vi "TestStand_Builder ( Test-Build ).vi"(8 "error out":errorcluster, 9 "Working_Dir":path, 10 "Test_ID":string="Test\r\n", 11 "Test_Case":string="\nPrecondition:\nPC_1. Wait.Sec(Delay=2) // Wait for Sec\n\nTestProcedure:\nTP_1. Wait.mSec(Delay=1000)  //Waits for ms\n\nReset:\nRST_1. Wait.Sec(Delay=2)  //Waits for sec\r\n") -> (0 "error out 2":errorcluster)   [LabVIEW 2018, in "TestStand_Control.lvlib"]
uses:
  TestStand_Control.lvlib
  Module_Controls/TestStand ( KWD_Info ).ctl
  XML_Library/XML.lvclass
  XML_Library/XML ( Clone and Append Single Input ).vi
  XML_Library/XML ( Set Node Value Single Input ).vi
  XML_Library/XML ( Set Node Value Multiple Inputs ).vi
  XML_Library/XML ( Delete Node Value Single Input ).vi
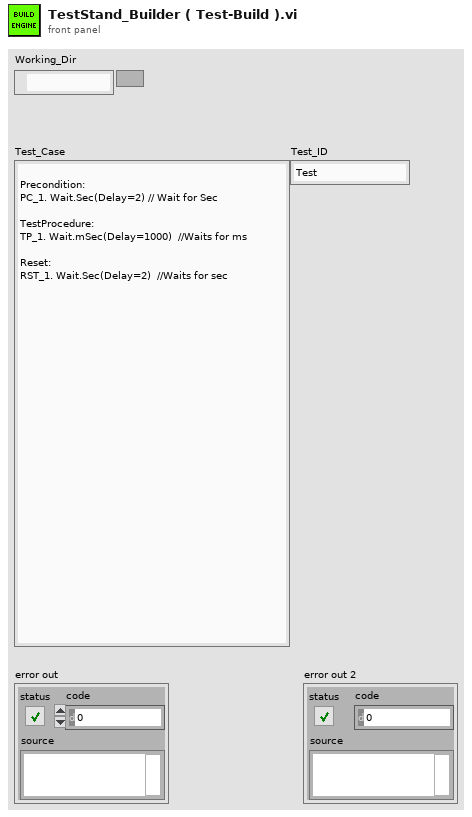
[diagram p1: front panel]
types:
  T1 = enum32{"Invalid", "Standard", "Closed", "Hidden", "Minimized", "Maximized"}
  T2 = enum32{"invalid app kind", "Development System", "Run Time System", "Student Edition", "Embedded LabVIEW", "Evaluation", "Custom"}
  T3 = typedef "TestStand ( KWD_Info ).ctl" = cluster{"Keyword_Name":string, "Keyword_Path":path, "Test_Case":string, "Test_Case Comment":string, "Kwd_Found":bool, "Keyword_Parameters":string}
  T4 = cluster{"Core":cluster{"Current VI Reference":refnum<vi>, "Close Panel on Exit?":bool}, "Test_Case":string, "Test_ID":string, "PreCondition":T3[], "TestProcedure":T3[], "Reset":T3[], "XML":refnum<class "XML.lvclass">}
  T5 = cluster{"Current VI Reference":refnum<vi>, "Close Panel on Exit?":bool}
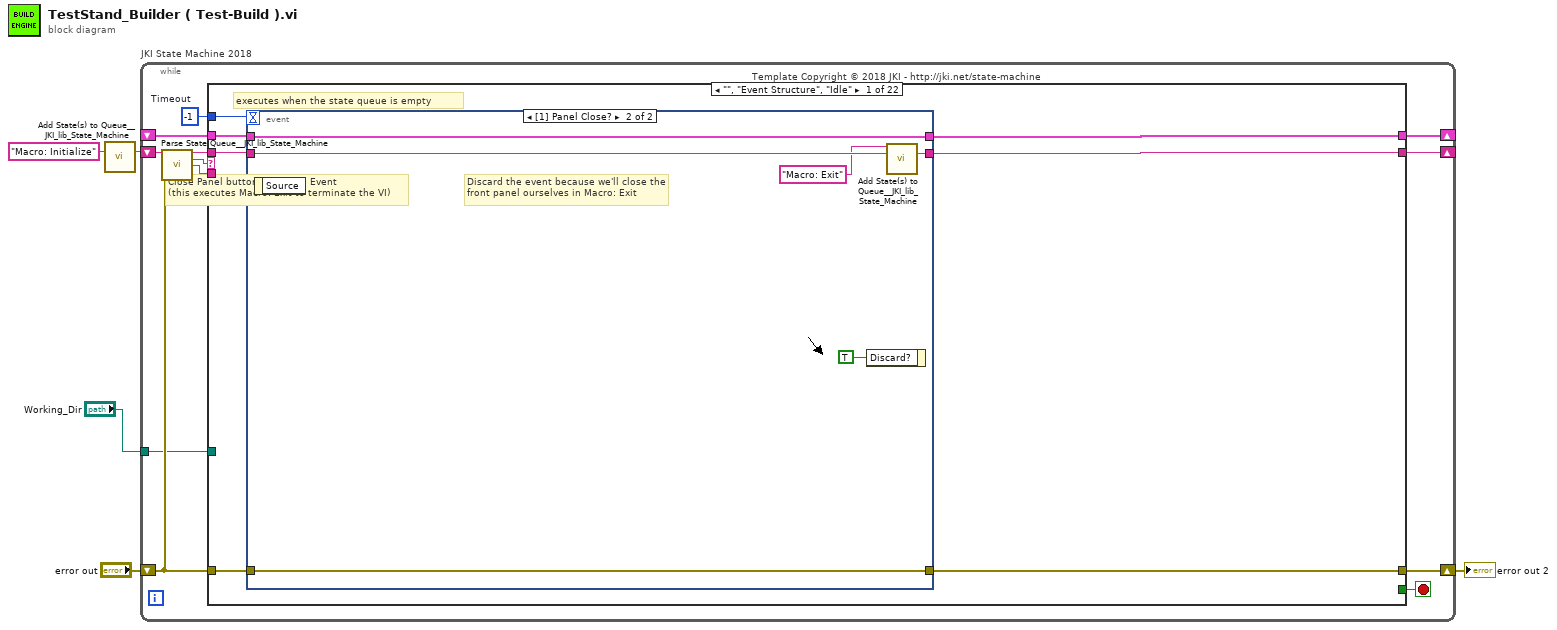
[diagram p0: block diagram]
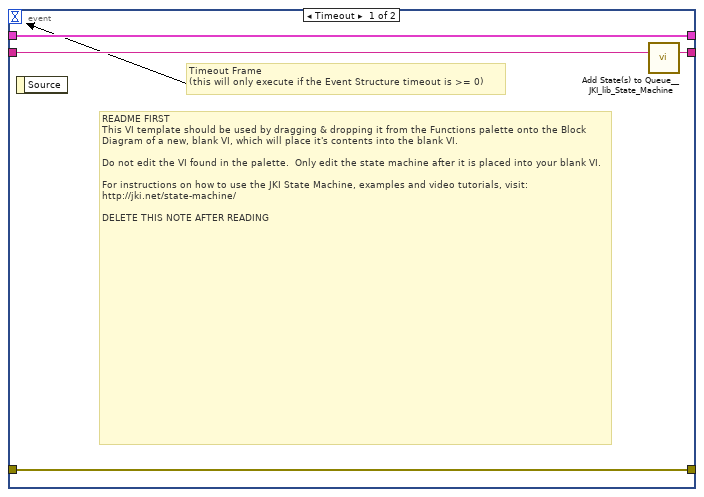
[diagram p2: hidden frame]
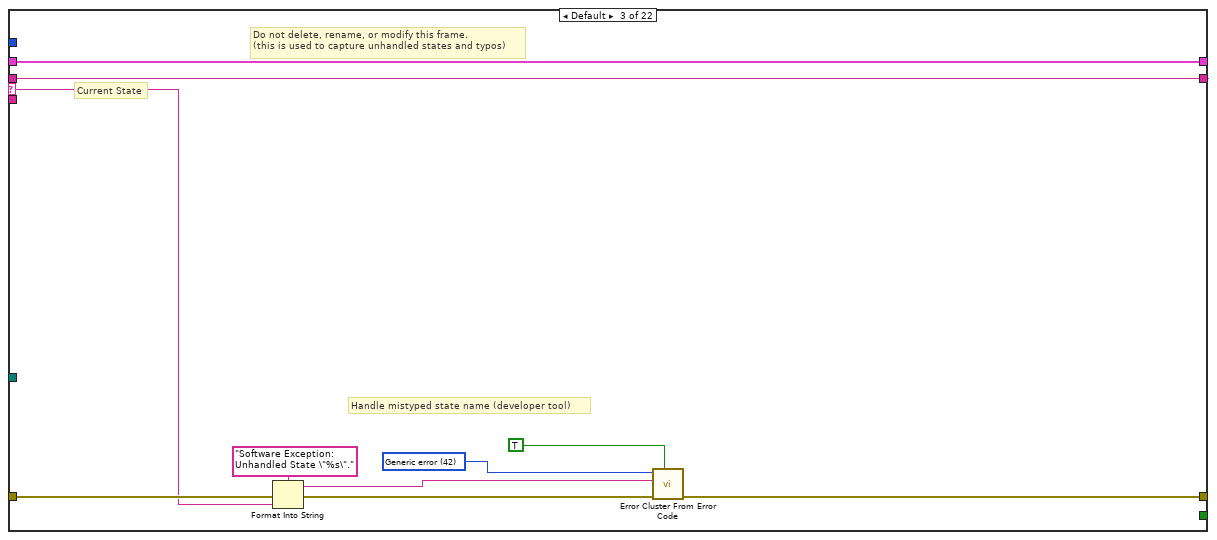
[diagram p4: hidden frame]
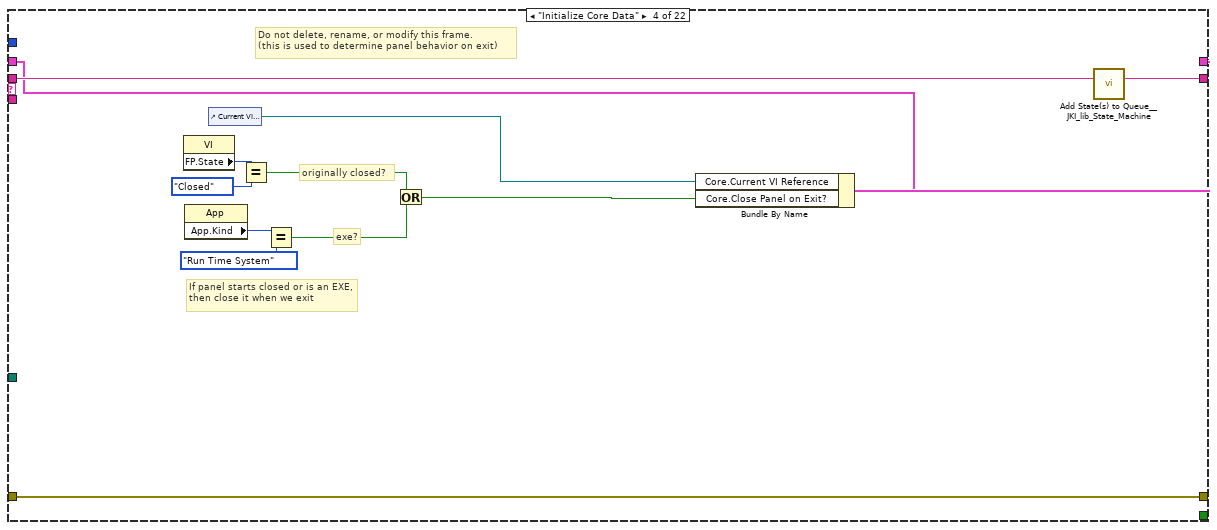
[diagram p5: hidden frame]
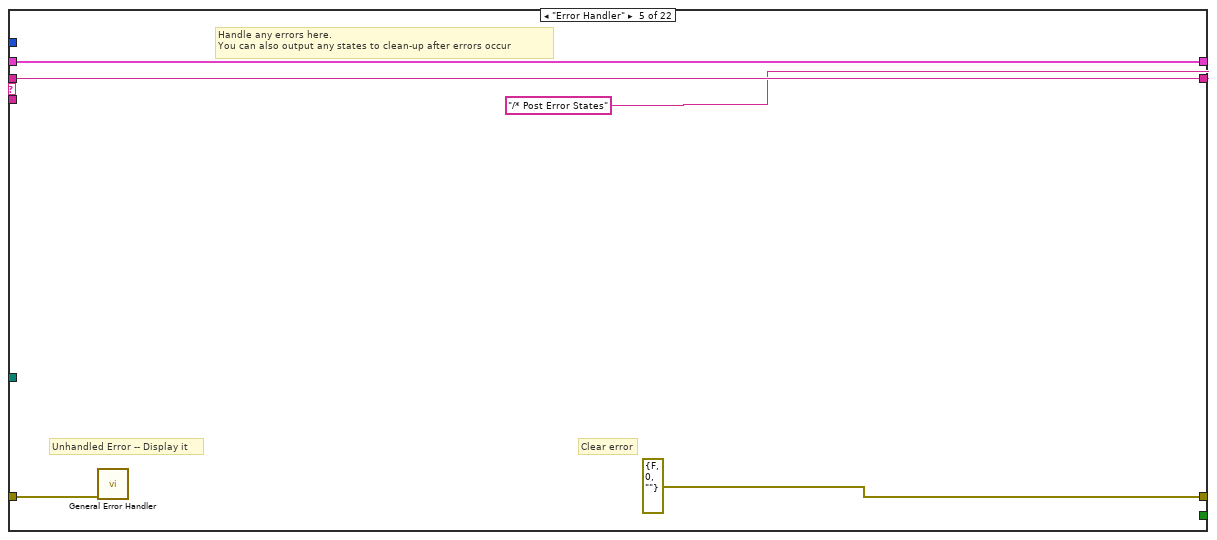
[diagram p6: hidden frame]
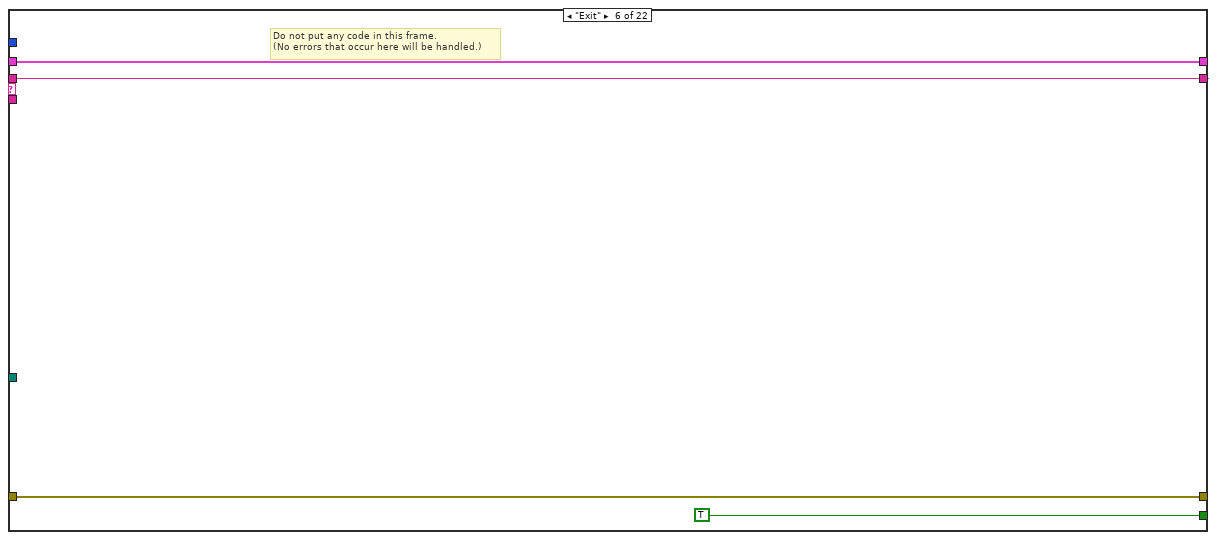
[diagram p7: hidden frame]
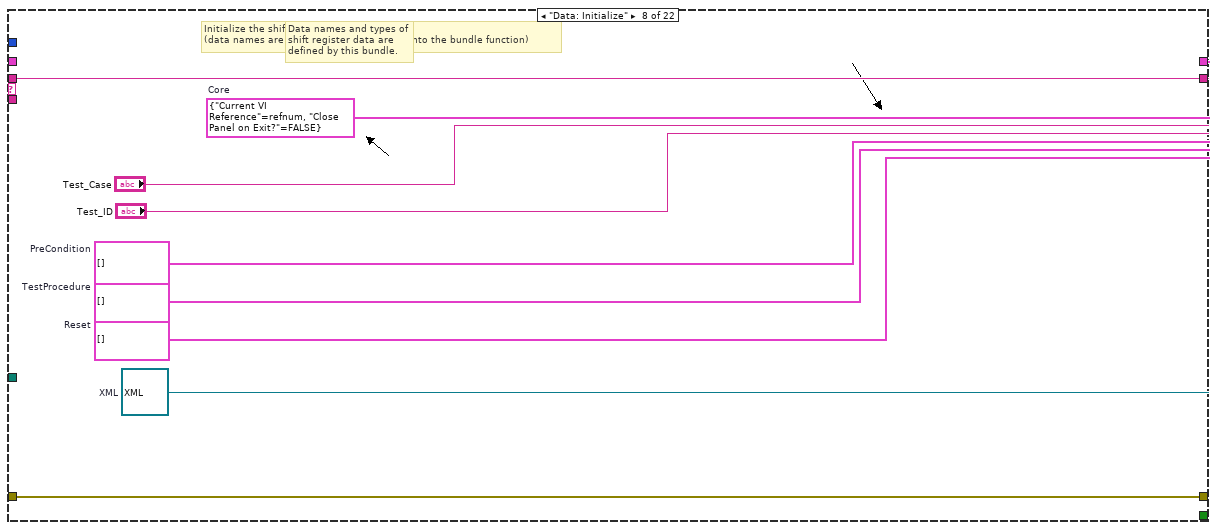
[diagram p9: hidden frame]
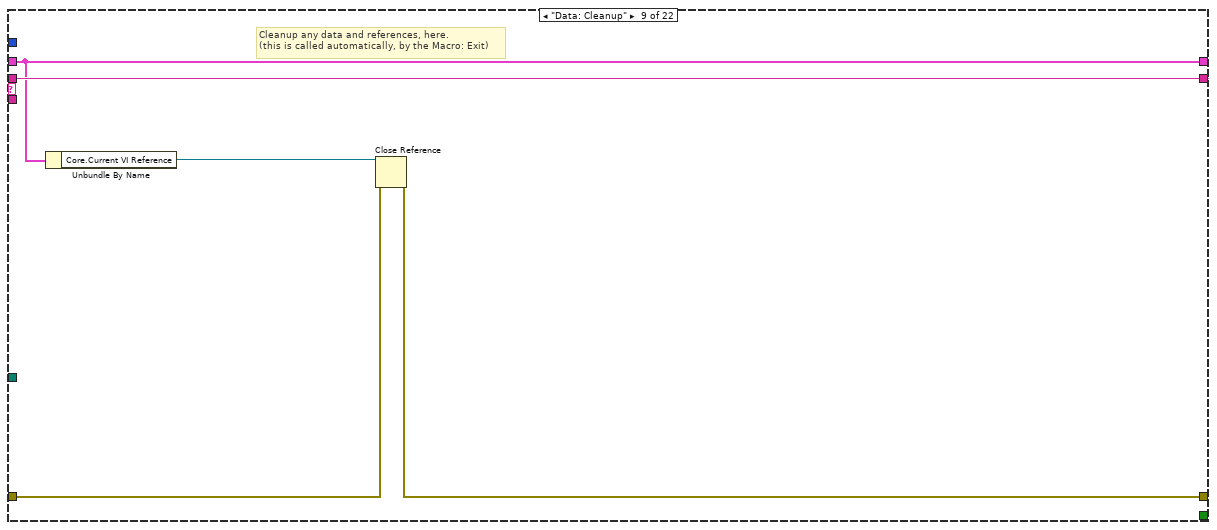
[diagram p10: hidden frame]
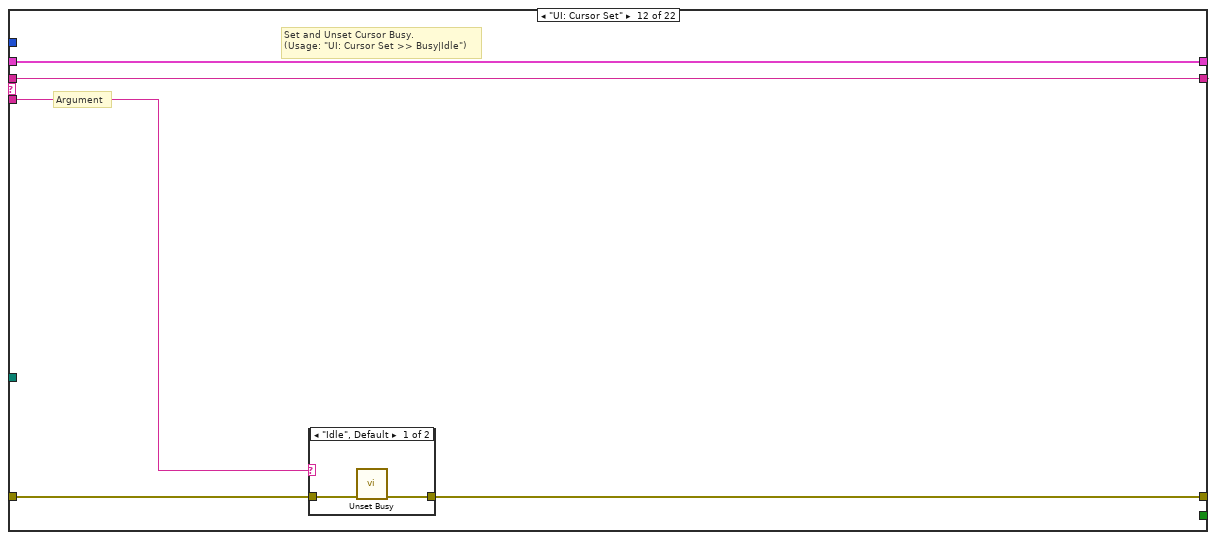
[diagram p13: hidden frame]
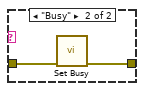
[diagram p14: hidden frame]
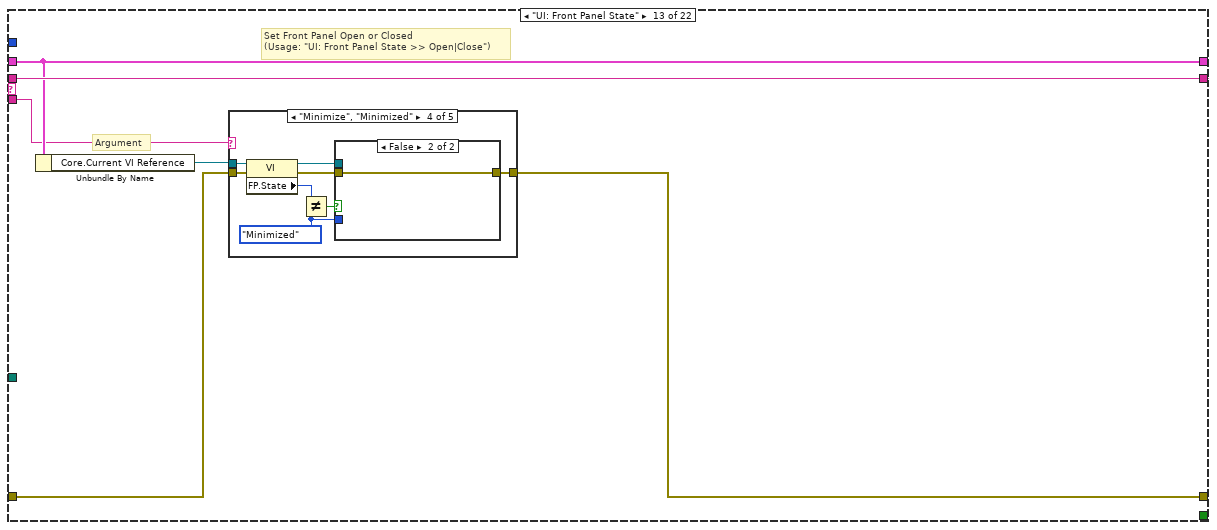
[diagram p15: hidden frame]
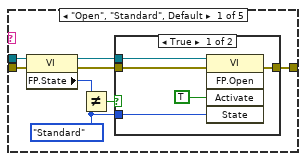
[diagram p16: hidden frame]
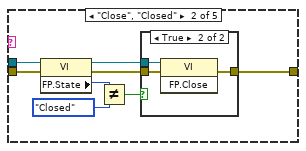
[diagram p18: hidden frame]
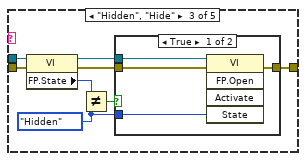
[diagram p20: hidden frame]
diagram:
  n1 = call <vilib>:"Add State(s) to Queue__JKI_lib_State_Machine.vi"("State(s) in (\"\")"="Macro: Initialize") -> ("States Out"=w5:string)  [unwired: 14 in]
  n2 = while "JKI State Machine 2018" {
    shift-right: [w10] -> _
    shift-left: _ -> [w9]
    shift-right: [w13] -> w2
    shift-left: "error out" -> [w7]
    shift-right: [w12] -> _
    shift-left: w5 -> [w14]
    tunnel: "Working_Dir" -> [w6]
    stop <- w11 stop-if-true
    w8 = -1  # Timeout
    # "Template Copyright © 2018 JKI - http://jki.net/state-machine"
    n3 = call <vilib>:"Parse State Queue__JKI_lib_State_Machine.vi"("State Queue"=w14, "Error In (no error)"=w7) -> ("Remaining States"=w16:string, "Current State"=w17:string, "Arguments"=w15:string)  [unwired: 11 in]
    n4 = case shown="\"\", \"Event Structure\", \"Idle\"" w17 {
      selector: w17 -> [_ _ w39 _ _ _ _ _ _ _ _ _ _ _ _ _ _ _ _ w241 _ _]
      tunnel: w16 -> [w24 w38 w43 w62 w68 w73 w77 w88 w94 w98 w102 w108 w119 w188 w193 w203 w207 w218 w230 w243 w344 w367]
      tunnel: w15 -> [_ _ _ _ _ _ _ _ _ _ _ w103 w113 _ _ _ _ _ _ _ _ _]
      tunnel: w9 -> [w22 w35 w41 w55 w65 w71 w74 _ w89 w95 w100 w106 w115 w185 w190 w200 w204 w214 w228 w238 w333 w363]
      tunnel: [w21 w36 w45 w59 errorcluster {"status"=FALSE, "code"=0, "source"=""} ("error out") w70 w75 w85 w90 w96 w99 w104 w116 w186 w191 w201 w205 w216 w225 w235 w324 w359] -> w13
      tunnel: w7 -> [w20 w36 w44 w59 w64 w70 w75 w85 w91 w96 w99 w105 w117 w186 w191 w201 w205 w216 w226 w236 w334 w360]
      tunnel: [w23 w37 w42 w61 w67 w72 w76 w87 w93 w97 w101 w107 w118 w187 w192 w202 w206 w217 w229 w242 w343 w366] -> w12
      tunnel: [_ _ _ _ _ TRUE _ _ _ _ _ _ _ _ _ _ _ _ _ _ _ _] -> w11
      tunnel: [w19 w35 w41 w60 w65 w71 w74 w86 w89 w95 w100 w106 w115 w185 w190 w200 w204 w213 w224 w233 w329 w363] -> w10
      tunnel: w8 -> [w18 _ _ _ _ _ _ _ _ _ _ _ _ _ _ _ _ _ _ _ _ _]
      tunnel: w6 -> [_ _ _ _ _ _ _ _ _ _ _ _ _ _ _ _ _ w208 w221 _ _ w356]
      frame "", "Event Structure", "Idle" {
        # "executes when the state queue is empty"
        n5 = event shown="[1] Panel Close?" {
          selector: _ -> [_ _]
          dyn-events: _ -> [_ _]
          timeout: w18 -> [_ _]
          tunnel: w24 -> [w28 w34]
          tunnel: [w27 w33] -> w23
          tunnel: w22 -> [w25 w31]
          tunnel: [w26 w32] -> w21
          tunnel: w20 -> [w26 w32]
          tunnel: [w25 w31] -> w19
          event Timeout {
            # "README FIRST\nThis VI template should be used by dragging & dropping it from the Functions palette onto the Block Diagram of a new, blank VI, which will place it's contents into the blank VI.\n\nDo not edit the VI found in the palette.  Only edit the state machine after it is placed into your blank VI.\n\nFor instructions on how to use the JKI State Machine, examples and video tutorials, visit:\nhttp://jki.net/state-machine/\n\nDELETE THIS NOTE AFTER READING"
            # "Timeout Frame\n(this will only execute if the Event Structure timeout is >= 0)"
            n6 = event-data() -> ()  [unwired: 1 in, 1 out]
            n7 = call <vilib>:"Add State(s) to Queue__JKI_lib_State_Machine.vi"("State(s) in (\"\")"=w28) -> ("States Out"=w27:string)  [unwired: 14 in]
          }
          event Panel Close? {
            # "Discard the event because we'll close the front panel ourselves in Macro: Exit"
            # "Close Panel button (pressed) Event\n(this executes Macro: Exit to terminate the VI)"
            n8 = event-data() -> ()  [unwired: 1 in, 1 out]
            n9 = event-data("Discard?"=TRUE) -> ()  [unwired: 1 in, 1 out]
            n10 = call <vilib>:"Add State(s) to Queue__JKI_lib_State_Machine.vi"("State(s) in Front (\"\")"="Macro: Exit", "State(s) in (\"\")"=w34) -> ("States Out"=w33:string)  [unwired: 13 in]
          }
        }
      }
      frame "---------- Core ----------" {
        # "Do not put any code in this frame.\n(it is a separator no-op)"
        n11 = call <vilib>:"Add State(s) to Queue__JKI_lib_State_Machine.vi"("State(s) in (\"\")"=w38) -> ("States Out"=w37:string)  [unwired: 14 in]
      }
      frame Default {
        w48 = 42 items=["No error", "Argument error", "Memory is full", "Out of zone", "End of file", "File already open", "Generic file I/O error", "File not found", "File permission error", "Disk is full", "Duplicate path", "Too many files open", "System feature not enabled", "Resource file not found", "Cannot add resource", "Resource not found", "Image not found", "Image memory error", "Pen does not exist", "Config type invalid", "Config token not found", "Config parse error", "Config memory error", "Bad external code format", "Bad external code offset", "External code not present", "Null window", "Destroy window error", "Null menu", "Print aborted", "Bad print record", "Print driver error", "Windows error during printing", "Memory error during printing", "Print dialog error", "Generic print error", "Invalid device refnum", "Device not found", "Device parameter error", "Device unit error", "Cannot open device", "Device call aborted", "Generic error", "Cancelled by user", "Object ID too low", "Object ID too high", "Object not in heap", "Unknown heap", "Unknown object (invalid DefProc)", "Unknown object (DefProc not in table)", "Message out of range", "Invalid (null) method", "Unknown message", "Manager call not supported", "Bad address", "Network operation in progress", "Network operation timed out", "Connection is busy", "Network attribute not supported", "Network error", "Address in use", "System out of memory", "Connection aborted", "Connection refused", "Not connected", "Already connected", "Connection closed", "Initialization error (interapplication manager)", "Bad occurrence", "Wait on unbound occurrence handler", "Occurrence queue overflow", "Datalog type conflict", "Unused", "Unrecognized type (interapplication manager)", "Memory corrupt", "Failed to make temporary DLL", "Old CIN version", "Drag socket not found", "Failed to load drop-object", "Failed to register OLE object", "Failed to release OLE object", "Format specifier type mismatch", "Unknown format specifier", "Too few format specifiers", "Too many format specifiers", "Scan failed", "Newer CIN version", "Error converting to variant", "Runtime menu error", "Password tampered", "Variant attribute not found", "Incompatible variant data type", "Event data is not available", "Event Store is not present", "Occurrence is not found", "Event Queue is not created", "Event info is not available", "Refnum passed is NULL", "Error retrieving Class GUID", "Error retrieving CoClass GUID", "Error retrieving TypeLib GUID.", "Bad built application magic bytes.", "Specific driver is different from the specific driver associated with the Logical Name.", "There is no session opened to the class driver.", "Max Error", "MAX - Error with config objects", "MAX - Error loading configuration", "MAX - Group not supported"]
        # "Current State"
        # "Do not delete, rename, or modify this frame.\n(this is used to capture unhandled states and typos)"
        # "Handle mistyped state name (developer tool)"
        n12 = Format Into String(format string="Software Exception: Unhandled State \"%s\"." ("message"), error in=w44, w39) -> (resulting string=w47:string, error out=w46:errorcluster)  [unwired: 1 in]
        n13 = call <vilib>:"Error Cluster From Error Code.vi"("show call chain? (False)"=TRUE, "error in (no error)"=w46, "error message (\"\")"=w47, "error code (0)"=w48) -> ("error out"=w45:errorcluster)  [unwired: 5 in]
        n14 = call <vilib>:"Add State(s) to Queue__JKI_lib_State_Machine.vi"("State(s) in (\"\")"=w43) -> ("States Out"=w42:string)  [unwired: 14 in]
      }
      frame "Initialize Core Data" {
        # "Do not delete, rename, or modify this frame.\n(this is used to determine panel behavior on exit)"
        # "originally closed?"
        # "exe?"
        # "If panel starts closed or is an EXE, then close it when we exit"
        n15 = property class="VI"() -> ("FP.State"=w52:T1)  [unwired: 2 in, 2 out]
        n16 = property class="App"() -> ("App.Kind"=w58:T2)  [unwired: 2 in, 2 out]
        n17 = control-ref of="Current VI Reference"() -> (w53:refnum<vi>)
        n18 = Equal?(x=w52, y=T1."Closed" ("Front Panel Window:State")) -> (x = y?=w50:bool)
        n19 = Equal?(x=w58, y=T2."Run Time System" ("Application:Kind")) -> (x = y?=w56:bool)
        n20 = Or(x=w50, y=w56) -> (x .or. y?=w54:bool)
        n21 = Bundle By Name(cluster=w55, "Core.Current VI Reference"=w53, "Core.Close Panel on Exit?"=w54) -> (w60:T4)
        n22 = call <vilib>:"Add State(s) to Queue__JKI_lib_State_Machine.vi"("State(s) in (\"\")"=w62) -> ("States Out"=w61:string)  [unwired: 14 in]
      }
      frame "Error Handler" {
        # "Unhandled Error -- Display it"
        # "Handle any errors here.\nYou can also output any states to clean-up after errors occur"
        # "Clear error"
        n23 = call <vilib>:"General Error Handler.vi"("error in (no error)"=w64) -> ()  [unwired: 10 in, 5 out]
        n24 = call <vilib>:"Add State(s) to Queue__JKI_lib_State_Machine.vi"("State(s) in Front (\"\")"="/* Post Error States", "State(s) in (\"\")"=w68) -> ("States Out"=w67:string)  [unwired: 13 in]
      }
      frame "Exit" {
        # "Do not put any code in this frame.\n(No errors that occur here will be handled.)"
        n25 = call <vilib>:"Add State(s) to Queue__JKI_lib_State_Machine.vi"("State(s) in (\"\")"=w73) -> ("States Out"=w72:string)  [unwired: 14 in]
      }
      frame "---------- Data ----------" {
        # "Do not put any code in this frame.\n(It is a separator no-op. You can make a copy of this frame to create a new Data frame)"
        n26 = call <vilib>:"Add State(s) to Queue__JKI_lib_State_Machine.vi"("State(s) in (\"\")"=w77) -> ("States Out"=w76:string)  [unwired: 14 in]
      }
      frame "Data: Initialize" {
        w80 = refnum<class "XML.lvclass"> refnum  # XML
        w81 = T3[] []  # Reset
        w82 = T3[] []  # TestProcedure
        w78 = T3[] []  # PreCondition
        w84 = T5 {"Current VI Reference"=refnum, "Close Panel on Exit?"=FALSE}  # Core
        # "Data names and types of shift register data are defined by this bundle."
        # "Initialize the shift-register data, here.\n(data names are defined by what you wire into the bundle function)"
        n27 = call <vilib>:"Add State(s) to Queue__JKI_lib_State_Machine.vi"("State(s) in (\"\")"=w88) -> ("States Out"=w87:string)  [unwired: 14 in]
        n28 = Bundle("Core"=w84, "Test_Case"="Test_Case", "Test_ID"="Test_ID", "PreCondition"=w78, "TestProcedure"=w82, "Reset"=w81, "XML"=w80) -> (w86:T4)  [unwired: 1 in]
      }
      frame "Data: Cleanup" {
        # "Cleanup any data and references, here.\n(this is called automatically, by the Macro: Exit)"
        n29 = Unbundle By Name(w89) -> ("Core.Current VI Reference"=w92:refnum<vi>)
        n30 = Close Reference(reference=w92, error in (no error)=w91) -> (error out=w90:errorcluster)
        n31 = call <vilib>:"Add State(s) to Queue__JKI_lib_State_Machine.vi"("State(s) in (\"\")"=w94) -> ("States Out"=w93:string)  [unwired: 14 in]
      }
      frame "---------- UI ----------" {
        # "Do not put any code in this frame.\n(It is a separator no-op. You can make a copy of this frame to create a new UI frame)"
        n32 = call <vilib>:"Add State(s) to Queue__JKI_lib_State_Machine.vi"("State(s) in (\"\")"=w98) -> ("States Out"=w97:string)  [unwired: 14 in]
      }
      frame "UI: Initialize" {
        # "Initialize the User Interface, here.\n(this is called automatically, by the Macro: Init)"
        n33 = call <vilib>:"Add State(s) to Queue__JKI_lib_State_Machine.vi"("State(s) in (\"\")"=w102) -> ("States Out"=w101:string)  [unwired: 14 in]
      }
      frame "UI: Cursor Set" {
        # "Argument"
        # "Set and Unset Cursor Busy.\n(Usage: \"UI: Cursor Set >> Busy|Idle\")"
        n34 = case shown="\"Idle\", Default" w103 {
          tunnel: w105 -> [w110 w112]
          tunnel: [w109 w111] -> w104
          frame "Idle", Default {
            n35 = call <vilib>:"Unset Busy.vi"("error in (no error)"=w110) -> ("error out"=w109:errorcluster)  [unwired: 10 in]
          }
          frame "Busy" {
            n36 = call <vilib>:"Set Busy.vi"("error in (no error)"=w112) -> ("error out"=w111:errorcluster)  [unwired: 9 in, 1 out]
          }
        }
        n37 = call <vilib>:"Add State(s) to Queue__JKI_lib_State_Machine.vi"("State(s) in (\"\")"=w108) -> ("States Out"=w107:string)  [unwired: 14 in]
      }
      frame "UI: Front Panel State" {
        # "Argument"
        # "Set Front Panel Open or Closed\n(Usage: \"UI: Front Panel State >> Open|Close\")"
        n38 = Unbundle By Name(w115) -> ("Core.Current VI Reference"=w114:refnum<vi>)
        n39 = case shown="\"Minimize\", \"Minimized\"" w113 {
          tunnel: w117 -> [w125 w140 w151 w164 w177]
          tunnel: [w127 w141 w153 w166 w179] -> w116
          tunnel: w114 -> [w126 w138 w152 w165 w178]
          frame "Open", "Standard", Default {
            w120 = T1."Standard" ("State")
            n40 = property class="VI"(reference=w126, error in=w125) -> (reference out=w123:refnum<vi>, error out=w124:errorcluster, "FP.State"=w122:T1)
            n41 = Not Equal?(x=w122, y=w120) -> (x != y?=w121:bool)
            n42 = case shown="True" w121 {
              tunnel: [w131 w133] -> w127
              tunnel: w124 -> [w130 w133]
              tunnel: w123 -> [w129 _]
              tunnel: w120 -> [w128 _]
              frame True {
                n43 = invoke class="VI" method="FP.Open"(reference=w129, error in=w130, "Activate"=TRUE, "State"=w128) -> (error out=w131:errorcluster)  [unwired: 1 in, 4 out]
              }
              frame False {
              }
            }
          }
          frame "Close", "Closed" {
            n44 = property class="VI"(reference=w138, error in=w140) -> (reference out=w137:refnum<vi>, error out=w139:errorcluster, "FP.State"=w135:T1)
            n45 = Not Equal?(x=w135, y=T1."Closed" ("Front Panel Window:State")) -> (x != y?=w134:bool)
            n46 = case shown="True" w134 {
              tunnel: [w142 w145] -> w141
              tunnel: w139 -> [w142 w144]
              tunnel: w137 -> [_ w143]
              frame False {
              }
              frame True {
                n47 = invoke class="VI" method="FP.Close"(reference=w143, error in=w144) -> (error out=w145:errorcluster)  [unwired: 1 in, 2 out]
              }
            }
          }
          frame "Hidden", "Hide" {
            w146 = T1."Hidden" ("State")
            n48 = property class="VI"(reference=w152, error in=w151) -> (reference out=w149:refnum<vi>, error out=w150:errorcluster, "FP.State"=w148:T1)
            n49 = Not Equal?(x=w148, y=w146) -> (x != y?=w147:bool)
            n50 = case shown="True" w147 {
              tunnel: [w157 w158] -> w153
              tunnel: w150 -> [w156 w158]
              tunnel: w149 -> [w155 _]
              tunnel: w146 -> [w154 _]
              frame True {
                n51 = invoke class="VI" method="FP.Open"(reference=w155, error in=w156, "State"=w154) -> (error out=w157:errorcluster)  [unwired: 2 in, 4 out]
              }
              frame False {
              }
            }
          }
          frame "Minimize", "Minimized" {
            w159 = T1."Minimized" ("State")
            n52 = property class="VI"(reference=w165, error in=w164) -> (reference out=w162:refnum<vi>, error out=w163:errorcluster, "FP.State"=w161:T1)
            n53 = Not Equal?(x=w161, y=w159) -> (x != y?=w160:bool)
            n54 = case shown="False" w160 {
              tunnel: [w170 w171] -> w166
              tunnel: w163 -> [w169 w171]
              tunnel: w162 -> [w168 _]
              tunnel: w159 -> [w167 _]
              frame True {
                n55 = invoke class="VI" method="FP.Open"(reference=w168, error in=w169, "State"=w167) -> (error out=w170:errorcluster)  [unwired: 2 in, 4 out]
              }
              frame False {
              }
            }
          }
          frame "Maximize", "Maximized" {
            w172 = T1."Maximized" ("State")
            n56 = property class="VI"(reference=w178, error in=w177) -> (reference out=w175:refnum<vi>, error out=w176:errorcluster, "FP.State"=w174:T1)
            n57 = Not Equal?(x=w174, y=w172) -> (x != y?=w173:bool)
            n58 = case shown="True" w173 {
              tunnel: [w183 w184] -> w179
              tunnel: w176 -> [w182 w184]
              tunnel: w175 -> [w181 _]
              tunnel: w172 -> [w180 _]
              frame True {
                n59 = invoke class="VI" method="FP.Open"(reference=w181, error in=w182, "State"=w180) -> (error out=w183:errorcluster)  [unwired: 2 in, 4 out]
              }
              frame False {
              }
            }
          }
        }
        n60 = call <vilib>:"Add State(s) to Queue__JKI_lib_State_Machine.vi"("State(s) in (\"\")"=w119) -> ("States Out"=w118:string)  [unwired: 14 in]
      }
      frame "---------- Macro ----------" {
        # "Do not put any code in this frame.\n(It is a separator no-op. You can make a copy of this frame to create a new Macro frame)"
        n61 = call <vilib>:"Add State(s) to Queue__JKI_lib_State_Machine.vi"("State(s) in (\"\")"=w188) -> ("States Out"=w187:string)  [unwired: 14 in]
      }
      frame "Macro: Initialize" {
        w189 = "Data: Initialize\nInitialize Core Data\nUI: Initialize\nUI: Front Panel State >> Minimize\nBuild_Engine: TestCase_KWD"  # Data: Initialize Initialize Core Data UI: Initialize UI: Front Panel State >> Minimize Build_Engine: TestCase_KWD
        # "Initialization Macro\n(This is called once, when the VI starts)"
        n62 = call <vilib>:"Add State(s) to Queue__JKI_lib_State_Machine.vi"("State(s) in Front (\"\")"=w189, "State(s) in (\"\")"=w193) -> ("States Out"=w192:string)  [unwired: 13 in]
      }
      frame "Macro: Exit" {
        # "Exit Macro\n(This is called once, when the VI exits)"
        n63 = Unbundle By Name(w200) -> ("Core.Close Panel on Exit?"=w199:bool)
        n64 = Select(t="UI: Front Panel State >> Close", s=w199, f="") -> (s? t:f=w196:string)
        n65 = call <vilib>:"Add State(s) to Queue__JKI_lib_State_Machine.vi"("State(s) in (\"\")"=w196, "State(s) at Back (\"\")"="Data: Cleanup\nExit") -> ("States Out"=w194:string)  [unwired: 13 in]
        n66 = call <vilib>:"Add State(s) to Queue__JKI_lib_State_Machine.vi"("State(s) in Front (\"\")"=w194, "State(s) in (\"\")"=w203) -> ("States Out"=w202:string)  [unwired: 13 in]
      }
      frame "---------- Build_Engine ----------" {
        # "Your code here.\n(You can make a copy of, or modify, this frame)"
        n67 = call <vilib>:"Add State(s) to Queue__JKI_lib_State_Machine.vi"("State(s) in (\"\")"=w207) -> ("States Out"=w206:string)  [unwired: 14 in]
      }
      frame "Build_Engine: TestCase_KWD" {
        # "Your code here.\n(You can make a copy of, or modify, this frame)"
        n68 = Unbundle By Name(w214) -> ("Test_Case"=w215:string)
        n69 = call "TestStand_Control ( Keyword_TestCase_Linkage ).vi"("Working_Directory"=w208, "Test_Case"=w215) -> ("Reset"=w210:T3[], "TestProcedure"=w211:T3[], "PreCondition"=w212:T3[])  [unwired: 7 in]
        n70 = Bundle By Name(cluster=w214, "PreCondition"=w212, "TestProcedure"=w211, "Reset"=w210) -> (w213:T4)
        n71 = call <vilib>:"Add State(s) to Queue__JKI_lib_State_Machine.vi"("State(s) in Front (\"\")"="Build_Engine: Init" ("State(s) in Front (\"\")"), "State(s) in (\"\")"=w218) -> ("States Out"=w217:string)  [unwired: 13 in]
      }
      frame "Build_Engine: Init" {
        # "Your code here.\n(You can make a copy of, or modify, this frame)"
        n72 = Unbundle By Name(w228) -> ("XML"=w227:refnum<class "XML.lvclass">)
        n73 = Build Path(base path=w221, name or relative path="Template\\Template.seq") -> (appended path=w219:path)
        n74 = call "XML ( Open ).vi"("error in (no error)"=w226, "XML document"=w219, "XML in"=w227) -> ("error out"=w225:errorcluster, "XML out"=w223:refnum<class "XML.lvclass">)  [unwired: 7 in]
        n75 = Bundle By Name(cluster=w228, "XML"=w223) -> (w224:T4)
        n76 = call <vilib>:"Add State(s) to Queue__JKI_lib_State_Machine.vi"("State(s) in Front (\"\")"="Build_Engine: Build_PC" ("State(s) in Front (\"\")"), "State(s) in (\"\")"=w230) -> ("States Out"=w229:string)  [unwired: 13 in]
      }
      frame "Build_Engine: Build_PC", "Build_Engine: Build_RST", "Build_Engine: Build_TP" {
        # "Your code here.\n(You can make a copy of, or modify, this frame)"
        n77 = case shown="\"Build_Engine: Build_PC\", Default" w241 {
          tunnel: w238 -> [w313 w317 w321]
          tunnel: [w312 w316 w320] -> w240
          tunnel: ["Setup" "Main" "Cleanup"] -> w239
          tunnel: ["Build_Engine: Build_TP" "Build_Engine: Build_RST" "Build_Engine: Build_PostBuild"] -> w231
          frame "Build_Engine: Build_PC", Default {
            n78 = Unbundle By Name(w313) -> ("PreCondition"=w312:T3[])
          }
          frame "Build_Engine: Build_TP" {
            n79 = Unbundle By Name(w317) -> ("TestProcedure"=w316:T3[])
          }
          frame "Build_Engine: Build_RST" {
            n80 = Unbundle By Name(w321) -> ("Reset"=w320:T3[])
          }
        }
        n81 = Unbundle By Name(w238) -> ("XML"=w237:refnum<class "XML.lvclass">)
        n82 = for {
          tunnel: w240 -> [w244] mode=indexing
          tunnel: w239 -> [w249]
          shift-right: [w245] -> w232
          shift-left: w237 -> [w248]
          shift-right: [w247] -> w234
          shift-left: w236 -> [w246]
          n83 = Unbundle By Name(w244) -> ("Keyword_Path"=w251:path)
          n84 = call <vilib>:"Get File Extension.vi"("file"=w251) -> ("lowercase file extension"=w250:string)  [unwired: 6 in, 4 out]
          n85 = case shown="\"seq\"" w250 {
            tunnel: w249 -> [_ w255]
            tunnel: w248 -> [w253 w259]
            tunnel: [w252 w258] -> w247
            tunnel: w246 -> [w252 w257]
            tunnel: [w253 w256] -> w245
            tunnel: w244 -> [_ w254]
            frame "False", Default {
            }
            frame "seq" {
              n86 = for {
                N: 5 -> [_]
                shift-right: [w265] -> w256
                shift-left: w259 -> [w266]
                shift-right: [w264] -> w258
                shift-left: w257 -> [w263]
                tunnel: w255 -> [w261]
                tunnel: w254 -> [w262]
                i -> [w267]
                n87 = case shown="0" w267 {
                  tunnel: w266 -> [w269 w277 w283 w293 w300 w307]
                  tunnel: [w269 w276 w284 w294 w301 w308] -> w265
                  tunnel: [w268 w275 w285 w295 w302 w309] -> w264
                  tunnel: w263 -> [w268 w274 w282 w292 w299 w306]
                  tunnel: w261 -> [_ w270 _ _ _ _]
                  tunnel: w262 -> [_ _ w281 w290 w297 w304]
                  frame Default {
                  }
                  frame 0 {
                    # "Clone"
                    n88 = Format Into String(format string="/a:teststandfileheader/a:Data/a:subprops/a:Seq/a:value/a:value/a:Sequence/a:subprops/a:%s/a:value", w270) -> (resulting string=w271:string)  [unwired: 2 in, 1 out]
                    n89 = call-poly "XML ( Clone and Append ).vi"("error in (no error)"=w274, "Parent_Node"=w271, "Clone_Node"="/a:teststandfileheader/a:Data/a:subprops/a:Seq/a:value/a:value/a:Sequence/a:subprops/a:Setup/a:value/a:value/a:Step[@name=\"SequenceCallTemplate\"]/..", "XML in"=w277) -> ("error out"=w275:errorcluster, "XML out"=w276:refnum<class "XML.lvclass">)  [unwired: 6 in]
                  }
                  frame 1 {
                    # "Update the File Path"
                    n90 = Unbundle By Name(w281) -> ("Keyword_Path"=w280:path)
                    n91 = Path To String(path=w280) -> (string=w279:string)
                    n92 = call-poly "XML ( Set Node Value ).vi"("error in (no error)"=w282, "Value"=w279, "XPath expression"="a:value/a:Step/a:subprops/a:TS/a:subprops/a:SData/a:subprops/a:SFPath/a:value/text()", "XML in"=w283) -> ("error out"=w285:errorcluster, "XML out"=w284:refnum<class "XML.lvclass">)  [unwired: 6 in]
                  }
                  frame 2 {
                    w287 = "\""
                    # "Update the Expr"
                    n93 = Unbundle By Name(w290) -> ("Keyword_Parameters"=w289:string)
                    n94 = call <vilib>:"Trim Whitespace.vi"("string"=w289) -> ("trimmed string"=w286:string)  [unwired: 1 in]
                    n95 = Concatenate Strings(w287, w286, w287) -> (w288:string)
                    n96 = call-poly "XML ( Set Node Value ).vi"("error in (no error)"=w292, "Value"=w288, "XPath expression"="a:value/a:Step/a:subprops/a:TS/a:subprops/a:SData/a:subprops/a:ActualArgs/a:subprops/a:DataInAsStringTabArray/a:subprops/a:Expr/a:value/text()", "XML in"=w293) -> ("error out"=w295:errorcluster, "XML out"=w294:refnum<class "XML.lvclass">)  [unwired: 6 in]
                  }
                  frame 3 {
                    # "Update the Step_Name"
                    n97 = Unbundle By Name(w297) -> ("Test_Case"=w296:string)
                    n98 = call-poly "XML ( Set Node Value ).vi"("error in (no error)"=w299, "Value"=w296, "XPath expression"="a:value/a:Step/@name", "XML in"=w300) -> ("error out"=w302:errorcluster, "XML out"=w301:refnum<class "XML.lvclass">)  [unwired: 6 in]
                  }
                  frame 4 {
                    # "Update the Comment"
                    n99 = Unbundle By Name(w304) -> ("Test_Case Comment"=w303:string)
                    n100 = call-poly "XML ( Set Node Value ).vi"("error in (no error)"=w306, "Value"=w303, "XPath expression"="a:value/a:Step/a:comment/text()", "XML in"=w307) -> ("error out"=w309:errorcluster, "XML out"=w308:refnum<class "XML.lvclass">)  [unwired: 6 in]
                  }
                }
              }
            }
          }
        }
        n101 = Bundle By Name(cluster=w238, "XML"=w232) -> (w233:T4)
        n102 = Merge Errors(w234, w236) -> (w235:errorcluster)
        n103 = call <vilib>:"Add State(s) to Queue__JKI_lib_State_Machine.vi"("State(s) in Front (\"\")"=w231, "State(s) in (\"\")"=w243) -> ("States Out"=w242:string)  [unwired: 13 in]
      }
      frame "Build_Engine: Build_PostBuild" {
        # "Your code here.\n(You can make a copy of, or modify, this frame)"
        n104 = Unbundle By Name(w333) -> ("PreCondition"=w339:T3[], "TestProcedure"=w338:T3[], "Reset"=w337:T3[])
        n105 = Unbundle By Name(w333) -> ("XML"=w332:refnum<class "XML.lvclass">)
        n106 = Array Size(array=w339) -> (size(s)=w342:i32)
        n107 = Array Size(array=w338) -> (size(s)=w341:i32)
        n108 = Array Size(array=w337) -> (size(s)=w340:i32)
        n109 = Build Array(w342, w341, w340) -> (w336:i32[])
        n110 = Decrement(x=w336) -> (x-1=w335:i32[])
        n111 = for {
          tunnel: w335 -> [w346] mode=indexing
          tunnel: [w345] -> w330 mode=indexing
          n112 = Number To Decimal String(number=w346) -> (decimal integer string=w351:string)  [unwired: 1 in]
          n113 = Equal?(x=w351, y="-1") -> (x = y?=w352:bool)
          n114 = Select(t="" ("y"), s=w352, f=w351) -> (s? t:f=w353:string)
          n115 = Concatenate Strings("[" ("string"), w353, "]" ("string")) -> (w345:string)
        }
        n116 = call-poly "XML ( Set Node Value ).vi"("error in (no error)"=w334, "Value"=w330, "XPath expression"=string[] ["/a:teststandfileheader/a:Data/a:subprops/a:Seq/a:value/a:value/a:Sequence/a:subprops/a:Setup/a:value/@ubound", "/a:teststandfileheader/a:Data/a:subprops/a:Seq/a:value/a:value/a:Sequence/a:subprops/a:Main/a:value/@ubound", "/a:teststandfileheader/a:Data/a:subprops/a:Seq/a:value/a:value/a:Sequence/a:subprops/a:Cleanup/a:value/@ubound"], "XML in"=w332) -> ("error out"=w325:errorcluster, "XML out"=w327:refnum<class "XML.lvclass">)  [unwired: 6 in]
        n117 = call-poly "XML ( Delete Node ).vi"("error in (no error)"=w325, "Child_Node"="/a:teststandfileheader/a:Data/a:subprops/a:Seq/a:value/a:value/a:Sequence/a:subprops/a:Setup/a:value/a:value/a:Step[@name=\"SequenceCallTemplate\"]/..", "Parent_Node"="/a:teststandfileheader/a:Data/a:subprops/a:Seq/a:value/a:value/a:Sequence/a:subprops/a:Setup/a:value", "XML in"=w327) -> ("error out"=w324:errorcluster, "XML out"=w326:refnum<class "XML.lvclass">)  [unwired: 6 in]
        n118 = Bundle By Name(cluster=w333, "XML"=w326) -> (w329:T4)
        n119 = call <vilib>:"Add State(s) to Queue__JKI_lib_State_Machine.vi"("State(s) in Front (\"\")"="Build_Engine: Close" ("State(s) in Front (\"\")"), "State(s) in (\"\")"=w344) -> ("States Out"=w343:string)  [unwired: 13 in]
      }
      frame "Build_Engine: Close" {
        # "Your code here.\n(You can make a copy of, or modify, this frame)"
        n120 = Build Path(base path=w356, name or relative path="TestBuilds") -> (appended path=w354:path)
        n121 = Unbundle By Name(w363) -> ("XML"=w361:refnum<class "XML.lvclass">, "Test_ID"=w362:string)
        n122 = Concatenate Strings(w362, ".seq" ("name or relative path")) -> (w364:string)
        n123 = Build Path(base path=w354, name or relative path=w364) -> (appended path=w358:path)
        n124 = call "XML ( Save ).vi"("error in (no error)"=w360, "Path"=w358, "XML in"=w361) -> ("error out"=w359:errorcluster)  [unwired: 7 in, 1 out]
        n125 = call <vilib>:"Add State(s) to Queue__JKI_lib_State_Machine.vi"("State(s) in Front (\"\")"="Macro: Exit" ("State(s) in Front (\"\")"), "State(s) in (\"\")"=w367) -> ("States Out"=w366:string)  [unwired: 13 in]
      }
    }
  }
  "error out 2" <- w2
